vi "Set Parameter.vi"(4 "RingText.Text":string, 6 "txtpower":dbl, 7 "txtstepwave":dbl, 8 "error in":errorcluster, 9 "txtstopwave":dbl, 10 "txtstartwave":dbl, 11 "Address Cluster":T1 {"tsl_communcation_method" items=["GPIB", "C232C", "TCPIP", "USB"]; "MPM_communcation_method" items=["GPIB", "C232C", "TCPIP", "USB"]}) -> (0 "error out":errorcluster, 3 "ILSTS":refnum<k24>)   [LabVIEW 2017]
uses:
  CTL/Address Cluster.ctl
  D:/test/ILSTS/LV_IL/LV_IL_Sample_x86/DLL/InstrumentDLL.dll
  DLL/InstrumentDLL.dll
  D:/test/ILSTS/LV_IL/LV_IL_Sample_x86/DLL/STSProcess.dll
  DLL/STSProcess.dll
  Share/PowerMonitorType.vi
  Share/Sweep_Speed.vi
  Share/Acctual_Step.vi
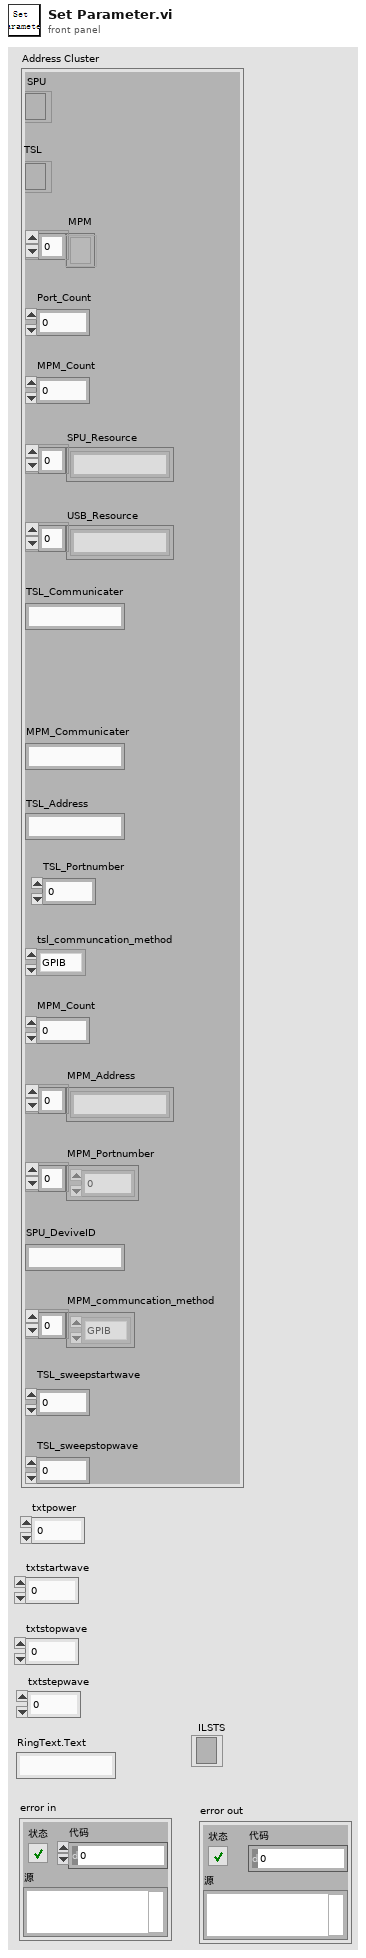
[diagram p1: front panel]
types:
  T1 = typedef "Address Cluster.ctl" = cluster{"SPU":refnum<k24>, "MPM":refnum<k24>[], "Port_Count":dbl, "MPM_Count":dbl, "SPU_Resource":string[], "USB_Resource":string[], "MPM_Communicater":string, "MPM_Count":dbl, "MPM_Address":string[], "MPM_Portnumber":dbl[], "SPU_DeviveID":string, "MPM_communcation_method":i32[], "TSL_sweepstartwave":dbl, "TSL_sweepstopwave":dbl, "TSL_Address":string, "TSL_Communicater":string, "TSL":refnum<k24>, "tsl_communcation_method":i32, "TSL_Portnumber":dbl}
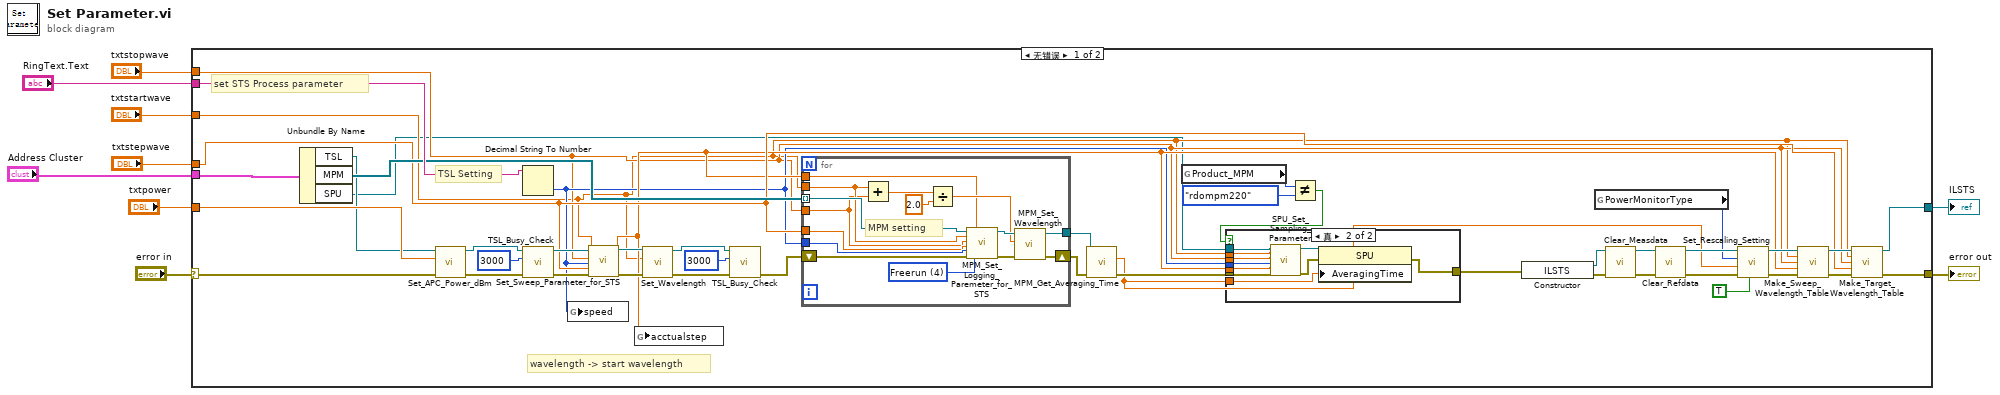
[diagram p0: block diagram]
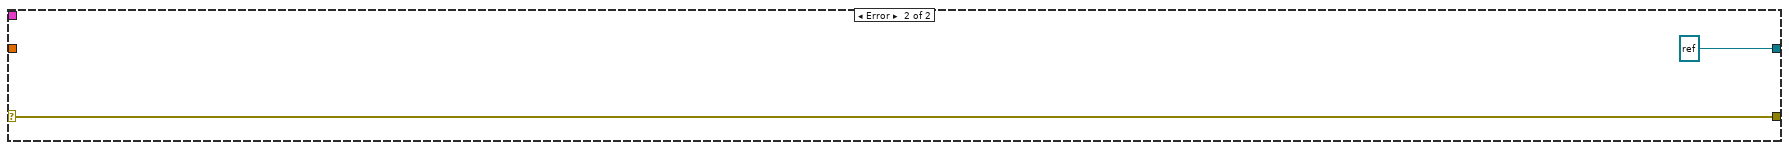
[diagram p3: hidden frame]
diagram:
  n1 = case shown="无错误" "error in" {
    selector: "error in" -> [w50 w82]
    tunnel: "txtstepwave" -> [w24 _]
    tunnel: "RingText.Text" -> [w54 _]
    tunnel: "txtpower" -> [w53 _]
    tunnel: [w23 refnum<k24> refnum ("STSProcess.ILSTS")] -> w1
    tunnel: "Address Cluster" -> [w51 _]
    tunnel: [w49 w82] -> w4
    tunnel: "txtstopwave" -> [w17 _]
    tunnel: "txtstartwave" -> [w16 _]
    frame No Error {
      # "set STS Process parameter"
      # "wavelength -> start wavelength"
      # "TSL Setting"
      n2 = Unbundle By Name(w51) -> ("TSL"=w30:refnum<k24>, "MPM"=w52:refnum<k24>[], "SPU"=w15:refnum<k24>)
      n3 = call "Set_APC_Power_dBm.vi"(".NET Reference in"=w30, "Setting Power"=w53, "error in (no error)"=w50) -> ("Reference out"=w47:refnum<k24>, "error out"=w48:errorcluster)  [unwired: 6 in]
      n4 = Decimal String To Number(string=w54) -> (number=w18:i32)  [unwired: 2 in, 1 out]
      n5 = call "TSL_Busy_Check.vi"("error in (no error)"=w48, "Wait time(msec)"=3000, ".NET Reference in"=w47) -> ("error out"=w45:errorcluster, "Reference out"=w44:refnum<k24>)  [unwired: 7 in]
      n6 = global write "Sweep_Speed.vi" "speed"(w18) -> ()
      n7 = call "Set_Sweep_Parameter_for_STS.vi"(".NET Reference in"=w44, "startwave"=w16, "stopwave"=w17, "speed"=w18, "rescalingstep"=w24, "error in (no error)"=w45) -> ("Reference out"=w43:refnum<k24>, "acctualstep"=w19:dbl, "error out"=w42:errorcluster)  [unwired: 11 in]
      n8 = global write "Acctual_Step.vi" "acctualstep"(w19) -> ()
      n9 = call "Set_Wavelength.vi"("error in (no error)"=w42, "txtsetwave"=w16, ".NET Reference in"=w43) -> ("error out"=w29:errorcluster, "Reference out"=w25:refnum<k24>)  [unwired: 3 in]
      n10 = call "TSL_Busy_Check.vi"("error in (no error)"=w29, "Wait time(msec)"=3000, ".NET Reference in"=w25) -> ("error out"=w28:errorcluster)  [unwired: 7 in, 1 out]
      n11 = for {
        tunnel: w52 -> [w80] mode=indexing
        tunnel: w16 -> [w71]
        tunnel: w17 -> [w70]
        tunnel: w18 -> [w78]
        tunnel: w24 -> [w76]
        shift-right: [w74] -> w31
        shift-left: w28 -> [w79]
        tunnel: [w73] -> w32
        tunnel: w19 -> [w66]
        w77 = 4 items=["ManualRangeConstant", "ManualRangeSweep", "AutoRangeConstant", "AutoRangeSweep", "Freerun"] ("mode")
        # "MPM setting"
        n12 = Add(x=w71, y=w70) -> (x+y=w69:dbl)
        n13 = Divide(x=w69, y=2.0) -> (x/y=w67:dbl)
        n14 = call "MPM_Set_Logging_Paremeter_for_STS.vi"(".NET Reference in"=w80, "startwave"=w71, "stopwave"=w70, "wavestep"=w76, "speed"=w78, "error in (no error)"=w79, "acctualstep"=w66, "mode"=w77) -> ("Reference out"=w72:refnum<k24>, "error out"=w75:errorcluster)  [unwired: 10 in]
        n15 = call "MPM_Set_Wavelength.vi"("error in (no error)"=w75, "Wavelength(nm)"=w67, ".NET Reference in"=w72) -> ("error out"=w74:errorcluster, "Reference out"=w73:refnum<k24>)  [unwired: 7 in]
      }
      n16 = call "MPM_Get_Averaging_Time.vi"("error in (no error)"=w31, ".NET Reference in"=w32) -> ("error out"=w20:errorcluster, "time out"=w11:dbl)  [unwired: 7 in, 1 out]
      n17 = global read "PowerMonitorType.vi" "Product_MPM"() -> (w14:enum32{"rdompm210", "rdompm220"})
      n18 = Not Equal?(x=w14, y=enum32{"rdompm210", "rdompm220"}."rdompm220") -> (x != y?=w12:bool)
      n19 = case shown="真" w12 {
        tunnel: w20 -> [w55 w65]
        tunnel: w19 -> [_ w64]
        tunnel: w18 -> [_ w63]
        tunnel: w17 -> [_ w62]
        tunnel: w16 -> [_ w61]
        tunnel: w15 -> [_ w60]
        tunnel: [w55 w56] -> w10
        tunnel: w11 -> [_ w57]
        frame False {
        }
        frame True {
          n20 = call "SPU_Set_Sampling_Parameter.vi"("引用"=w60, "startwave"=w61, "stopwave"=w62, "speed"=w63, "triggerstep"=w64, "错误输入（无错误）"=w65) -> ("引用输出"=w59:refnum<k24>, "error IO"=w58:errorcluster)  [unwired: 12 in]
          n21 = property class="SPU"(reference=w59, error in=w58, "AveragingTime"=w57) -> (error out=w56:errorcluster)  [unwired: 1 out]
        }
      }
      n22 = constructor class="ILSTS"(error in=w10) -> (reference out=w26:refnum<k24>, error out=w22:errorcluster)  [unwired: 2 in, 1 out]
      n23 = global read "PowerMonitorType.vi" "PowerMonitorType"() -> (w21:enum16{"DAQ", "MPM_220", "TSL_LOGG"})
      n24 = call "Clear_Measdata.vi"("error in (no error)"=w22, ".NET Reference in"=w26) -> ("error out"=w40:errorcluster, "Reference out"=w41:refnum<k24>)  [unwired: 8 in]
      n25 = call "Clear_Refdata.vi"("error in (no error)"=w40, ".NET Reference in"=w41) -> ("error out"=w38:errorcluster, "Reference out"=w39:refnum<k24>)  [unwired: 8 in]
      n26 = call "Set_Rescaling_Setting.vi"("isOriginalMonitor"=TRUE, "error in (no error)"=w38, "avg"=w11, "PowerMonitorType"=w21, ".NET Reference in"=w39) -> ("error out"=w35:errorcluster, "Reference out"=w36:refnum<k24>)  [unwired: 5 in]
      n27 = call "Make_Sweep_Wavelength_Table.vi"(".NET Reference in"=w36, "startwave"=w16, "endwave"=w17, "triggerstep"=w19, "error in (no error)"=w35) -> ("Reference out"=w34:refnum<k24>, "error out"=w33:errorcluster)  [unwired: 9 in]
      n28 = call "Make_Target_Wavelength_Table.vi"(".NET Reference in"=w34, "startwave"=w16, "endwave"=w17, "targetdatastep"=w24, "error in (no error)"=w33) -> ("Reference out"=w23:refnum<k24>, "error out"=w49:errorcluster)  [unwired: 9 in]
    }
    frame Error {
    }
  }
  "error out" <- w4
  "ILSTS" <- w1
